vi "XY Graph Update Plot & Style.vi"(4 "Y Array":dbl[](array[numeric]), 6 "X Array":dbl[](array[numeric]), 8 "Error In":errorcluster, 9 "XY Plot Style in":T1={"Plot Index"=-1, "Plot.Bar Plot Style"=0, "Plot.DigitalLineStyle"=0, "Plot.TransitionLocation"=0, "Plot.Transition Type"=0, "Plot.Fill To"=0, "Plot.Fill/Pt. Color"=0, "Plot.Label Format"=0, "Plot.Line Style"=0, "Plot.Line Width"=0, "Plot.Plot Color"=0, "Plot.Plot Interpolation"=0, "Plot.Plot Name"="", "Plot.Point Style"=0, "Plot.Visible?"=FALSE, "Plot.XScaleIdx"=0, "Plot.YScaleIdx"=0, "Plot.Anti-aliased"=FALSE}, 10 "Plot Idx":i32, 11 "XY Graph refnum":refnum<vi>) -> (0 "Error Out":errorcluster, 1 "Plot Style out":T1, 3 "Plot Name":string)   [LabVIEW 2021, in "XY Graph Add-Ons.lvlib"]
uses:
  XY Graph Add-Ons.lvlib
  XY Graph Plot Properties.ctl
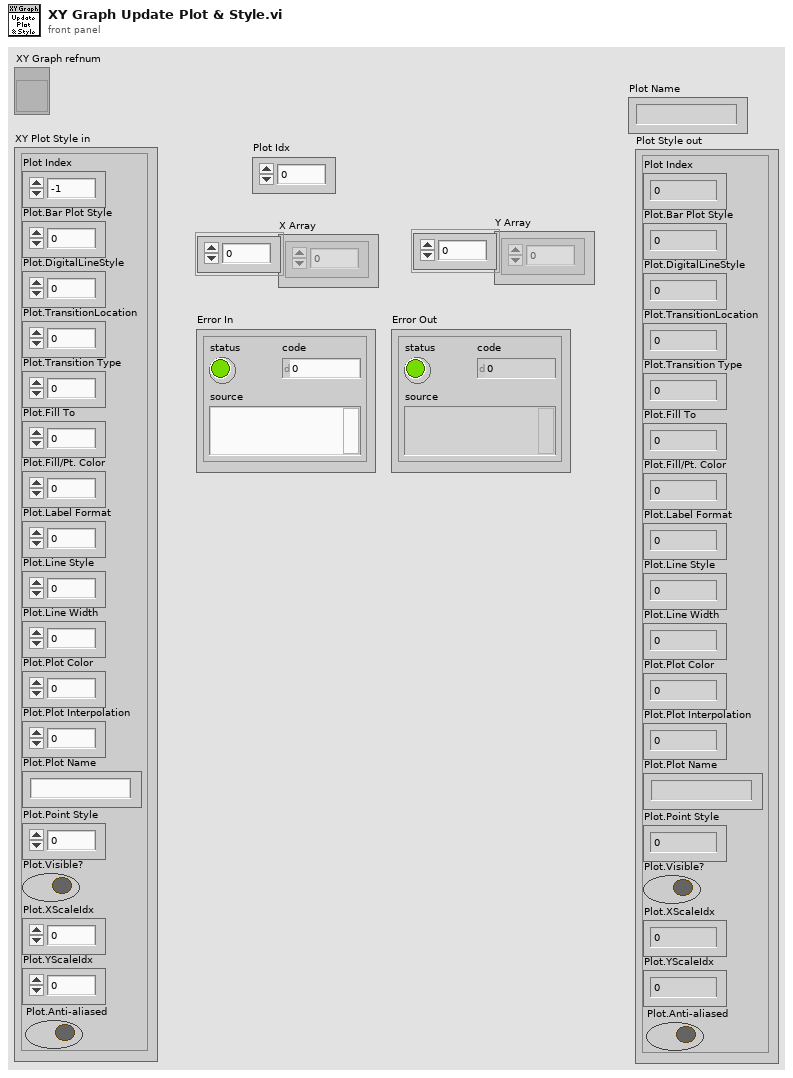
[diagram p1: front panel]
types:
  T1 = typedef "XY Graph Add-Ons.lvlib/XY Graph Plot Properties.ctl" = cluster{"Plot Index":i32, "Plot.Bar Plot Style":u8, "Plot.DigitalLineStyle":u8, "Plot.TransitionLocation":u8, "Plot.Transition Type":u8, "Plot.Fill To":i16, "Plot.Fill/Pt. Color":u32, "Plot.Label Format":u8, "Plot.Line Style":u8, "Plot.Line Width":u8, "Plot.Plot Color":u32, "Plot.Plot Interpolation":u8, "Plot.Plot Name":string, "Plot.Point Style":u8, "Plot.Visible?":bool, "Plot.XScaleIdx":u32, "Plot.YScaleIdx":u32, "Plot.Anti-aliased":bool}
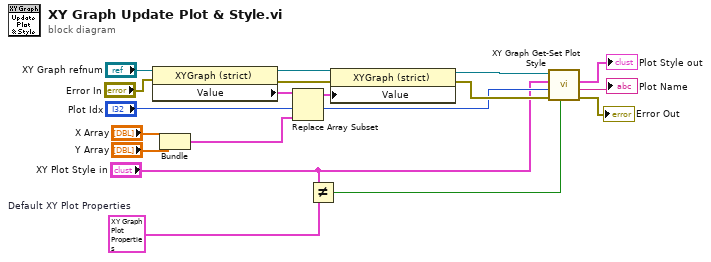
[diagram p0: block diagram]
diagram:
  w4 = T1 {"Plot Index"=-1, "Plot.Bar Plot Style"=0, "Plot.DigitalLineStyle"=0, "Plot.TransitionLocation"=0, "Plot.Transition Type"=0, "Plot.Fill To"=0, "Plot.Fill/Pt. Color"=0, "Plot.Label Format"=0, "Plot.Line Style"=0, "Plot.Line Width"=0, "Plot.Plot Color"=0, "Plot.Plot Interpolation"=0, "Plot.Plot Name"="", "Plot.Point Style"=0, "Plot.Visible?"=FALSE, "Plot.XScaleIdx"=0, "Plot.YScaleIdx"=0, "Plot.Anti-aliased"=FALSE}  # Default XY Plot Properties
  n1 = property class="XYGraph (strict)"(reference="XY Graph refnum", error in="Error In") -> (reference out=w13:refnum<vi>, error out=w12:errorcluster, "Value"=w17:cluster{"X Array":dbl[], "Y Array":dbl[]}[])
  n2 = Bundle("X Array"="X Array", "Y Array"="Y Array") -> (w14:cluster{"X Array":dbl[], "Y Array":dbl[]})  [unwired: 1 in]
  n3 = Replace Array Subset(array=w17, new element=w14, index="Plot Idx") -> (w11:cluster{"X Array":dbl[], "Y Array":dbl[]}[])
  n4 = Not Equal?(x="XY Plot Style in", y=w4) -> (x != y?=w2:bool)
  n5 = property class="XYGraph (strict)"(reference=w13, error in=w12, "Value"=w11) -> (reference out=w10:refnum<vi>, error out=w9:errorcluster)
  n6 = call "XY Graph Get-Set Plot Style.vi"("Get (F)/Set"=w2, "Error In"=w9, "Plot Index"="Plot Idx", "Plot Style in"="XY Plot Style in", "XYGraph in"=w10) -> ("Error Out"=→"Error Out":errorcluster, "Plot Name"=→"Plot Name":string, "Plot Style out"=→"Plot Style out":T1)  [unwired: 3 in, 1 out]
